vi "Init Data.vi"(8 "error in (no error)":errorcluster, 10 "Data Object":refnum<class "Factory Plugin Framework.lvclass">=refnum, 11 "Protocol Interface in":refnum<class "Protocol Interface.lvclass">) -> (0 "error out":errorcluster, 3 "Protocol Interface out":refnum<class "Protocol Interface.lvclass">)   [LabVIEW 2018, in "Protocol Interface.lvlib" / "Protocol Interface.lvclass"]
uses:
  Protocol Interface.lvclass
  FPF.lvlibp/Factory Plugin Framework.lvclass
  Protocol Interface.lvclass/Protocol Interface.ctl
  Read Pattern Script.vi
  Read Protocol Type.vi
  Read Num of cycle Rd.vi
  Read Period(ms).vi
  Read Wait(ms).vi
  Write Pattern Script.vi
  Write Protocol Type.vi
  Write Num of cycle Rd.vi
  Write Period(ms).vi
  Write Wait(ms).vi
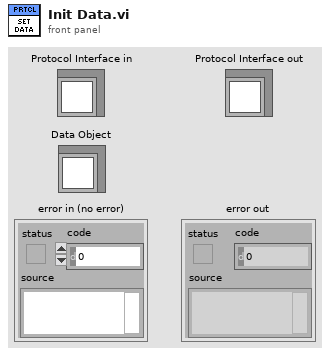
[diagram p1: front panel]
types:
  T1 = typedef "Protocol Type.ctl" = enum16{"BML_LS", "BML_HS", "SPI_3W", "SPI_4W"}
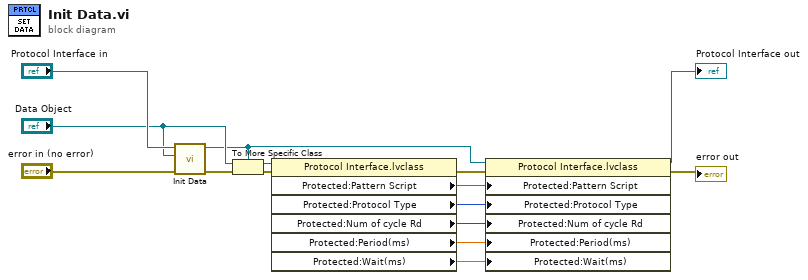
[diagram p0: block diagram]
diagram:
  n1 = call-parent "Init Data.vi"("error in (no error)"="error in (no error)", "Data Object"="Data Object", "Factory Plugin Framework in"="Protocol Interface in") -> ("error out"=w14:errorcluster, "Factory Plugin Framework out"=w4:refnum<class "Protocol Interface.lvclass">)  [unwired: 7 in]
  n2 = To More Specific Class(target class=w4, reference="Data Object", error in=w14) -> (specific class reference=w11:refnum<class "Protocol Interface.lvclass">, error out=w10:errorcluster)
  n3 = property class="Protocol Interface.lvclass"(reference=w11, error in=w10) -> (error out=w9:errorcluster, "Protected:Pattern Script"=w8:string, "Protected:Protocol Type"=w7:T1, "Protected:Num of cycle Rd"=w3:u32, "Protected:Period(ms)"=w2:dbl, "Protected:Wait(ms)"=w1:dbl)  [unwired: 1 out]
  n4 = property class="Protocol Interface.lvclass"(reference=w4, error in=w9, "Protected:Pattern Script"=w8, "Protected:Protocol Type"=w7, "Protected:Num of cycle Rd"=w3, "Protected:Period(ms)"=w2, "Protected:Wait(ms)"=w1) -> (reference out=→"Protocol Interface out":refnum<class "Protocol Interface.lvclass">, error out=→"error out":errorcluster)
